vi "WriteModeDM.vi"(5 "ClearV":bool, 9 "Amplitudes":dbl[](array[numeric]), 10 "Modes":i32[](array[numeric]), 11 "Device":i32) -> (3 "Voltage Map":dbl[][](array[numeric]))   [LabVIEW 2015]
uses:
  <vilib>/Analysis/baseanly.llb/A x Vector.vi
  <vilib>/Analysis/NI_AALBase.lvlib
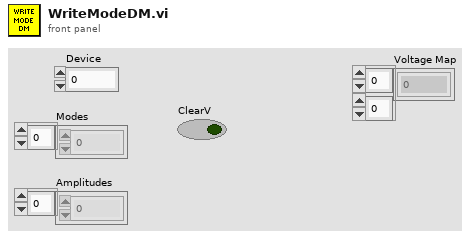
[diagram p1: front panel]
types:
  T1 = typedef "NI_Matrix.lvlib/RealMatrix.ctl" = dbl[][]
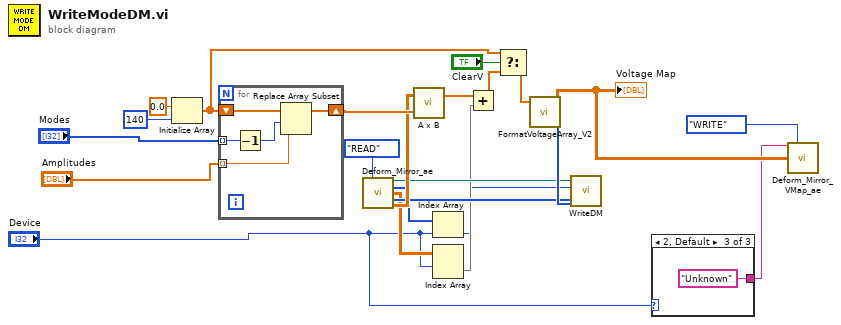
[diagram p0: block diagram]
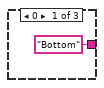
[diagram p2: hidden frame]
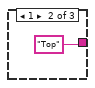
[diagram p3: hidden frame]
diagram:
  n1 = Initialize Array(0.0 ("element"), 140 ("dimension size")) -> (w1:dbl[])
  n2 = for {
    tunnel: "Modes" -> [w27] mode=indexing
    tunnel: "Amplitudes" -> [w25] mode=indexing
    shift-right: [w24] -> w21
    shift-left: w1 -> [w28]
    n3 = Decrement(x=w27) -> (x-1=w26:i32)
    n4 = Replace Array Subset(array=w28, new element=w25, index=w26) -> (w24:dbl[])
  }
  n5 = call "Deform_Mirror_ae.vi"("Enum"=enum16{"WRITE", "READ"}."READ") -> ("Refnum Out"=w14:refnum<k7>, "IDs Out"=w12:i32[], "Flat Files Out"=w11:dbl[][], "Multi Map Data Out"=w13:i32[], "Mode Matrix Out"=w15:T1)  [unwired: 10 in]
  n6 = call-poly <vilib>:"A x B.vi"("Vector"=w21, "A"=w15) -> ("A x Vector"=w16:dbl[])  [unwired: 1 out]
  n7 = Index Array(array=w12, index="Device") -> (element=w7:i32)
  n8 = Index Array(array=w11, index (row)="Device") -> (element=w10:dbl[])  [unwired: 1 in]
  n9 = Add ("Add.vi")(x=w16, y=w10) -> (x+y=w3:dbl[])
  n10 = Select(t=w1, s="ClearV", f=w3) -> (s? t:f=w2:dbl[])
  n11 = call "FormatVoltageArray_V2.vi"("Array in"=w2) -> ("Mirror Array"=w17:u16[], "Voltage Map"=w9:dbl[][])  [unwired: 9 in]
  "Voltage Map" <- w9
  n12 = call "WriteDM.vi"("reference in"=w14, "nDevId"=w7, "MultiDM  Mapping"=w13, "Voltage Array in"=w17) -> ()  [unwired: 2 in, 2 out]
  n13 = case shown="2, Default" "Device" {
    tunnel: ["Bottom" "Top" "Unknown"] -> w6
    frame 0 {
    }
    frame 1 {
    }
    frame 2, Default {
    }
  }
  n14 = call "Deform_Mirror_VMap_ae.vi"("Mirror ID"=w6, "Enum"=enum16{"WRITE", "READ"}."WRITE", "V Map In"=w9) -> ()  [unwired: 12 in, 1 out]
